vi "Manipulator Inertia Torque (Trajectory).vi"(8 "error in (no error)":errorcluster, 9 "joint acceleration trajectory":dbl[][](array[numeric]), 10 "joint position trajectory":dbl[][](array[numeric]), 11 "serial arm in":refnum<class "NI_Robotics_Serial Robot Arm.lvclass">) -> (0 "error out":errorcluster, 2 "torque trajectory":dbl[][](array[numeric]), 3 "serial arm out":refnum<class "NI_Robotics_Serial Robot Arm.lvclass">)   [LabVIEW 2017, in "NI_Kinematics.lvlib"]
doc: "Calculates the joint torques that result from inertia given the joint accelerations you specify. Wire data to the <B>joint positions</B> input to determine the polymorphic instance to use or manually select the instance.\n\n<B>.m file:</B> itorque"
uses:
  <vilib>/robotics/Kinematics/NI_Kinematics.lvlib
  <vilib>/robotics/Kinematics/Robot/NI_Robotics_Serial Robot Arm.lvclass
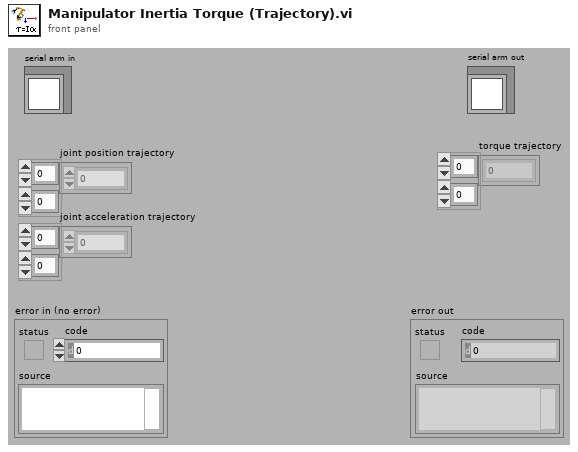
[diagram p1: front panel]
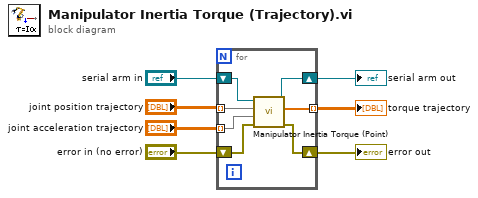
[diagram p0: block diagram]
diagram:
  n1 = for {
    tunnel: "joint position trajectory" -> [w12] mode=indexing
    tunnel: "joint acceleration trajectory" -> [w11] mode=indexing
    tunnel: [w10] -> w3 mode=indexing
    shift-right: [w8] -> w1
    shift-left: "error in (no error)" -> [w9]
    shift-right: [w13] -> w6
    shift-left: "serial arm in" -> [w14]
    n2 = call <vilib>:"Manipulator Inertia Torque (Point).vi"("error in (no error)"=w9, "joint accelerations"=w11, "joint positions"=w12, "serial arm in"=w14) -> ("error out"=w8:errorcluster, "torques"=w10:dbl[], "serial arm out"=w13:refnum<class "NI_Robotics_Serial Robot Arm.lvclass">)  [unwired: 5 in]
  }
  "serial arm out" <- w6
  "torque trajectory" <- w3
  "error out" <- w1
